vi "Shift distance data insert.vi"(8 "error in (no error)":errorcluster, 11 "移位距离":dbl) -> (0 "error out":errorcluster)   [LabVIEW 2016, in "AIRMAR WeatherCaster.lvlib"]
uses:
  AIRMAR WeatherCaster.lvlib
  <vilib>/addons/database/Auxilliary.llb/DB Tools Column Info.ctl
  <vilib>/addons/database/Auxilliary.llb/DB Tools DataTypes.ctl
  <vilib>/addons/database/NI_Database_API.lvlib
  <vilib>/Utility/VariantDataType/VariantType.lvlib
panel:
  in  "data in":cluster{"时间":timestamp, "移位距离":dbl}
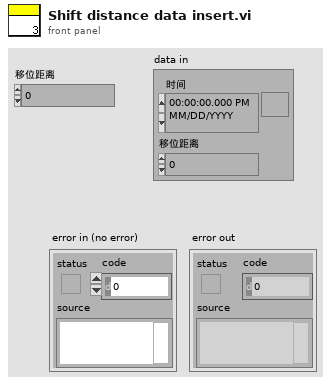
[diagram p1: front panel]
types:
  T1 = typedef "NI_Database_API.lvlib/DB Tools Column Info.ctl" = cluster{"column name":string, "data type":T2, "size":i32, "allow null?":bool}
  T2 = typedef "NI_Database_API.lvlib/DB Tools DataTypes.ctl" = enum16{"String", "Long (I32)", "Single (SGL)", "Double (DBL)", "Date/Time", "Binary"}
  T3 = typedef "VariantType.lvlib/Type.ctl" = enum8{"Invalid Type", "Void", "I8", "I16", "I32", "I64", "U8", "U16", "U32", "U64", "Single Float", "Double Float", "Extended Float", "Single Complex", "Double Complex", "Extended Complex", "Enum U8", "Enum U16", "Enum U32", "Enum U64", "Single Float With Unit", "Double Float With Unit", "Extended Float With Unit", "Single Complex with Unit", "Double Complex with Unit", "Extended Complex with Unit", "Boolean", "String", "Path", "Picture", "Tag", "Array", "Cluster", "Variant", "LV Variant", "Waveform", "Timestamp", "Digital Waveform", "Digital Data", "ExpressData", "Refnum", "External Data", "VI", "Poly VI", "LabVIEW Class Instance", "Fixed Point"}
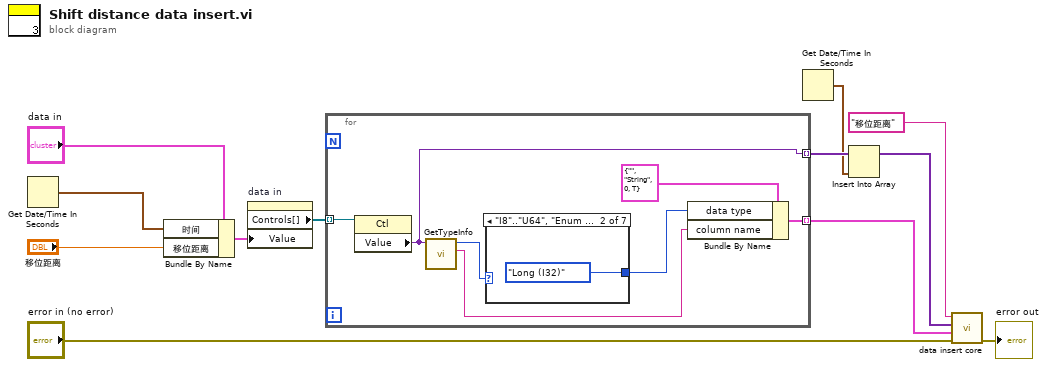
[diagram p0: block diagram]
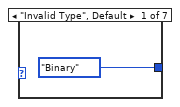
[diagram p2: hidden frame]
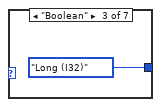
[diagram p3: hidden frame]
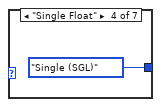
[diagram p4: hidden frame]
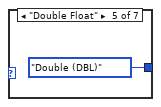
[diagram p5: hidden frame]
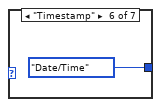
[diagram p6: hidden frame]
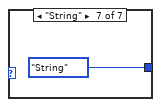
[diagram p7: hidden frame]
diagram:
  n1 = Get Date/Time In Seconds() -> (seconds since 1Jan1904=w3:timestamp)
  n2 = Bundle By Name(cluster="data in", "时间"=w3, "移位距离"="移位距离") -> (w2:cluster{"时间":timestamp, "移位距离":dbl})
  n3 = property on="data in" class="Clust (严格)"("Value"=w2) -> ("Controls[]"=w12:refnum<vi>[])  [unwired: 2 in, 2 out]
  n4 = for {
    tunnel: w12 -> [w19] mode=indexing
    tunnel: [w13] -> w11 mode=indexing
    tunnel: [w14] -> w6 mode=indexing
    n5 = property class="Ctl"(reference=w19) -> ("Value"=w13:variant)  [unwired: 1 in, 2 out]
    n6 = call <vilib>:"GetTypeInfo.vi"("Variant"=w13) -> ("Name"=w17:string, "Type Enum"=w16:T3)  [unwired: 6 in, 3 out]
    n7 = case shown="\"I8\"..\"U64\", \"Enum U8\"..\"Enum U64\"" w16 {
      tunnel: [DB_Tools_DataTypes."Binary" ("data type") DB_Tools_DataTypes."Long (I32)" ("data type") DB_Tools_DataTypes."Long (I32)" ("data type") DB_Tools_DataTypes."Single (SGL)" ("data type") DB_Tools_DataTypes."Double (DBL)" ("data type") DB_Tools_DataTypes."Date/Time" ("data type") DB_Tools_DataTypes."String" ("data type")] -> w15
      frame "Invalid Type", Default {
      }
      frame "I8".."U64", "Enum U8".."Enum U64" {
      }
      frame "Boolean" {
      }
      frame "Single Float" {
      }
      frame "Double Float" {
      }
      frame "Timestamp" {
      }
      frame "String" {
      }
    }
    n8 = Bundle By Name(cluster=T1 {"column name"="", "data type"=enum."String", "size"=0, "allow null?"=TRUE} ("column information"), "data type"=w15, "column name"=w17) -> (w14:T1)
  }
  n9 = Get Date/Time In Seconds() -> (seconds since 1Jan1904=w10:timestamp)
  n10 = Insert Into Array(array=w11, new element=w10) -> (w9:variant[])  [unwired: 1 in]
  n11 = call "data insert core.vi"("error in (no error)"="error in (no error)", "column information"=w6, "data"=w9, "table"="移位距离") -> ("error out"=→"error out":errorcluster)  [unwired: 7 in]
